vi "R2_Control.vi"() -> ()   [LabVIEW 2016]
uses:
  R2 Reactor Status v1.ctl
  Reactor Control/R1R2/R2/R2 SBR Mode Control.ctl
  Reactor Control/R1R2/R2/R2 pH Manual Control.ctl
  Reactor Control/R1R2/R2/R2 Pump Manual Control.ctl
  R2 DO Manual Control.ctl
  Reactor Control/R1R2/R2/R2Variables.lvlib
panel:
  out "Elapsed Time":dbl
  in  "Aerobic DO Control":T1={"DO set point (mg/L)"=1.5, "N2 Gain"=5.0, "Air Gain"=5.0, "DO Tolerance (mg/L)"=0.05, "Air Short Reaction Time (s)"=15.0, "Long Reaction Time (s)"=30.0, "N2 Short Reaction Time (s) 2"=10.0}
  out "pH and DO":cluster{"pH":dbl, "DO (mg/L)":dbl}(graph)
  out "DO Intercept":dbl
  out "DO Slope":dbl
  out "pH Intercept":dbl
  out "pH Slope":dbl
  in  "DO Control":T2
  in  "Reactor 2 Pumps Manual Control":T3
  in  "pH Control":T4
  in  "pH Control":T5={" pH Set Point"=7.5, " pH Tolerance"=0.1, "Reaction Time (s)"=15.0, "Pump On Time (s)"=3.0}
  in  "SBR Timing":T6={"Anaerobic Feed"=60.0, "Aerobic"=240.0, "Settle 1"=3.0, "Decant 1"=0.5, "Mix 2"=1.0, "Floc Effluent"=3.0, "Aerobic no DO control "=2.0, "Settle 2 (min)"=2.0, "Decant 2"=0.5, "Mix 3"=1.0, "Settle 3"=1.0, "Decant 3"=1.0, "Floc Return"=0.0}
  out "N2 and Air Flow":cluster{"N2 Flow":dbl, "Air Flow":dbl}(graph)
  out "Reactor 2 Status":T7 {"Compressed Air" format="%#.0g"; "Release Flow" format="%#.0g"; "DO Amp (A)" format="%#.4g"; "pH Amp (A)" format="%#.4g"; "DO (mg/L)" format="%#.2g"; "pH" format="%#.2g"}
  in  "Pumps Manual Control":bool
  in  "DO Manual Control":bool
  in  "pH Manual Control":bool
  in  "DO Calibrate":bool
  in  "pH Calibrate":bool
  # "On: Manual Mode\nOff: SBR Mode"
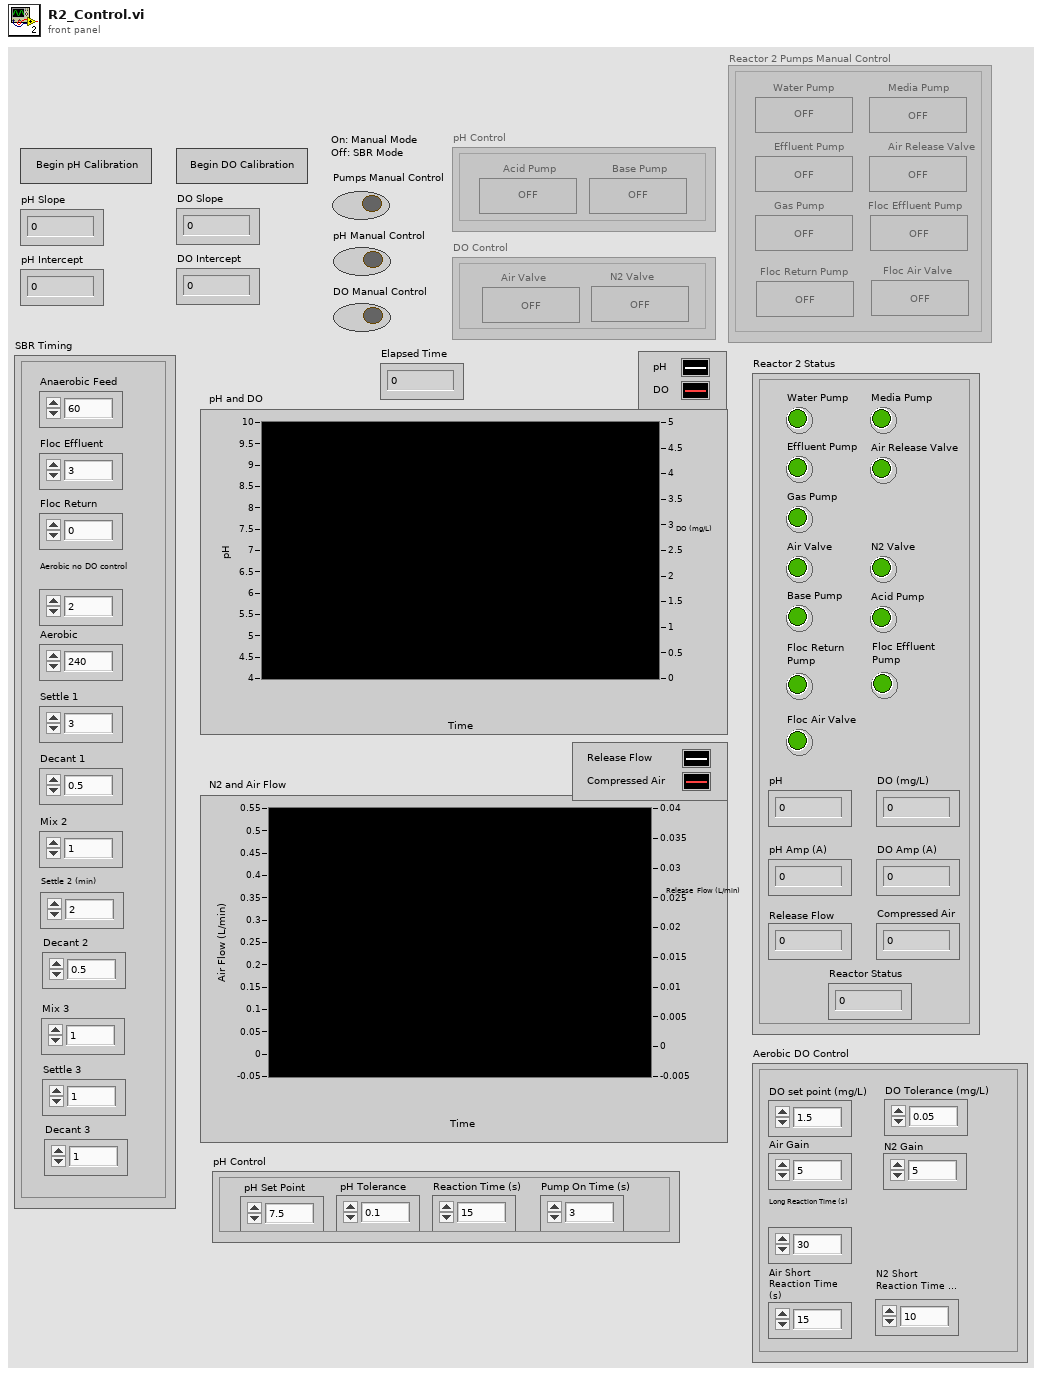
[diagram p1: front panel]
types:
  T1 = cluster{"DO set point (mg/L)":dbl, "N2 Gain":dbl, "Air Gain":dbl, "DO Tolerance (mg/L)":dbl, "Air Short Reaction Time (s)":dbl, "Long Reaction Time (s)":dbl, "N2 Short Reaction Time (s) 2":dbl}
  T2 = typedef "R2Variables.lvlib/R2 DO Manual Control.ctl" = cluster{"Air Valve":bool, "N2 Valve":bool}
  T3 = typedef "R2Variables.lvlib/R2 Pump Manual Control.ctl" = cluster{"Water Pump":bool, "Effluent Pump":bool, "Media Pump":bool, "Gas Pump":bool, "Air Release Valve":bool, "Floc Effluent Pump":bool, "Floc Return Pump":bool, "Floc Air Valve":bool}
  T4 = typedef "R2Variables.lvlib/R2 pH Manual Control.ctl" = cluster{"Acid Pump":bool, "Base Pump":bool}
  T5 = cluster{" pH Set Point":dbl, " pH Tolerance":dbl, "Reaction Time (s)":dbl, "Pump On Time (s)":dbl}
  T6 = typedef "R2Variables.lvlib/R2 SBR Mode Control.ctl" = cluster{"Anaerobic Feed":dbl, "Aerobic":dbl, "Settle 1":dbl, "Decant 1":dbl, "Mix 2":dbl, "Floc Effluent":dbl, "Aerobic no DO control ":dbl, "Settle 2 (min)":dbl, "Decant 2":dbl, "Mix 3":dbl, "Settle 3":dbl, "Decant 3":dbl, "Floc Return":dbl}
  T7 = typedef "R2Variables.lvlib/R2 Reactor Status v1.ctl" = cluster{"Water Pump":bool, "Media Pump":bool, "Effluent Pump":bool, "Base Pump":bool, "Gas Pump":bool, "Acid Pump":bool, "Air Release Valve":bool, "N2 Valve":bool, "pH":dbl, "DO (mg/L)":dbl, "pH Amp (A)":dbl, "DO Amp (A)":dbl, "Release Flow":dbl, "Compressed Air":dbl, "Reactor Status":sgl, "Air Valve":bool, "Floc Return \nPump":bool, "Floc Effluent\nPump ":bool, "Floc Air Valve":bool}
  T8 = enum8{"Enabled", "Disabled", "Disabled and Grayed Out"}
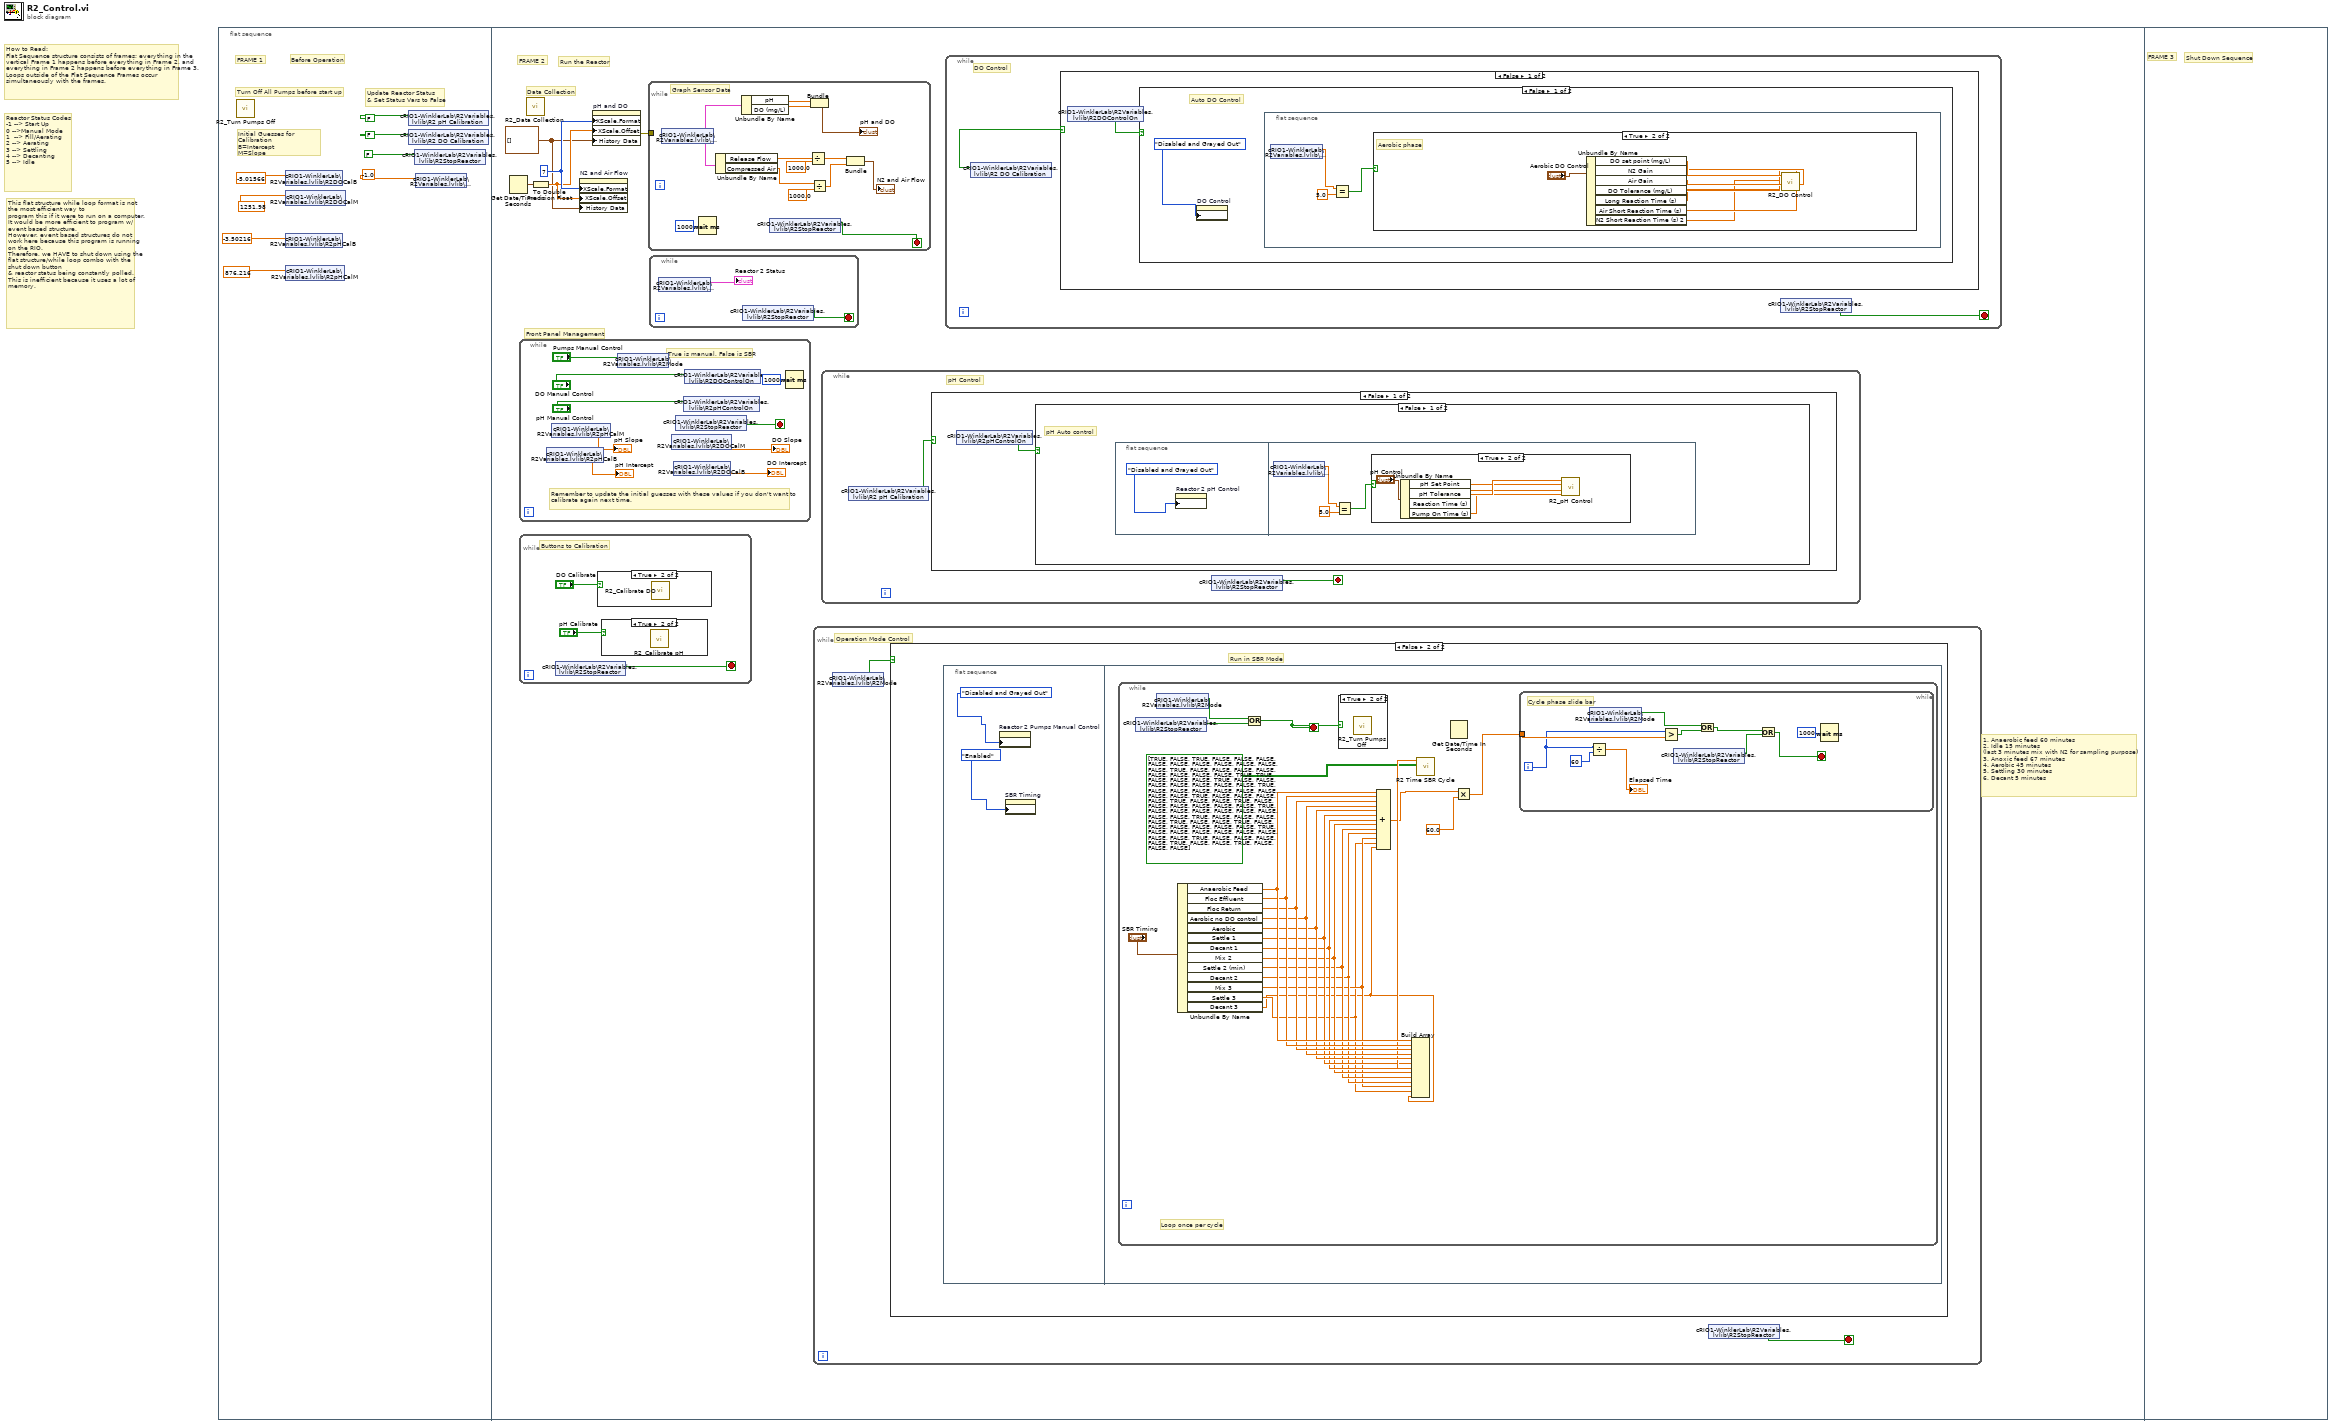
[diagram p0: block diagram]
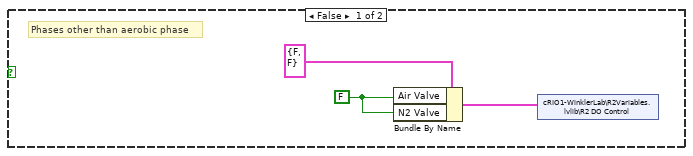
[diagram p2: hidden frame]
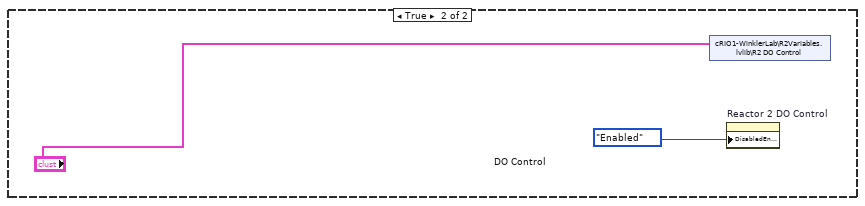
[diagram p3: hidden frame]
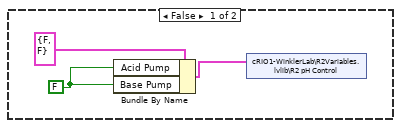
[diagram p7: hidden frame]
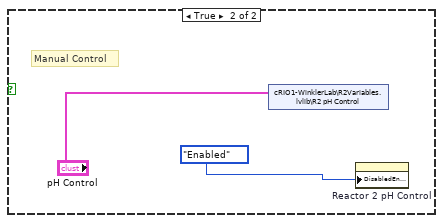
[diagram p8: hidden frame]
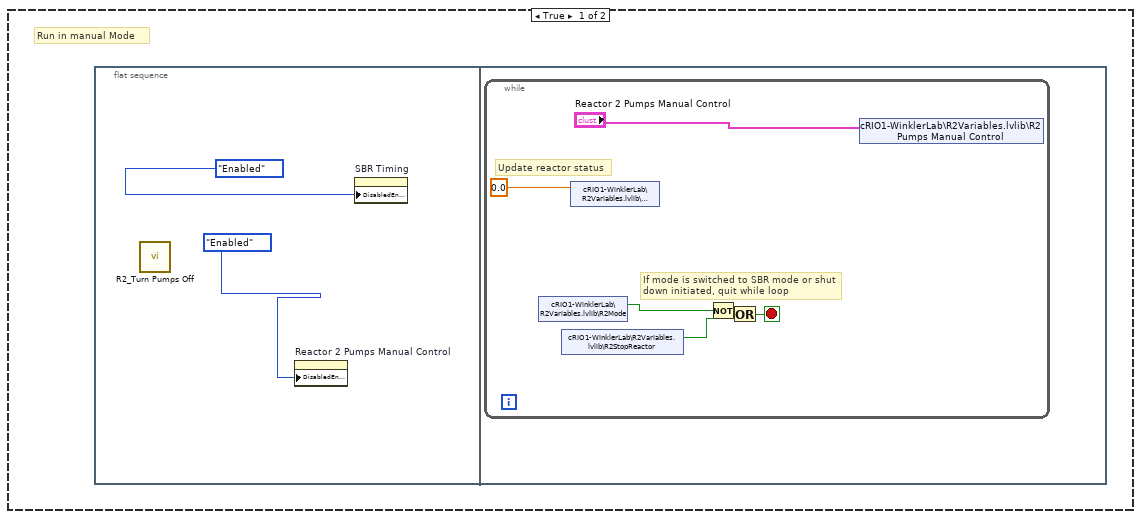
[diagram p10: hidden frame]
diagram:
  # "Reactor Status Codes\n-1 --> Start Up\n0 -->Manual Mode\n1  --> Fill/Aerating\n2 --> Aerating\n3 --> Settling\n4 --> Decanting\n5 --> Idle"
  # "How to Read:\nFlat Sequence structure consists of frames; everything in the vertical Frame 1 happens before everything in Frame 2, and everything in Frame 2 happens before everything in Frame 3.\nLoops outside of the Flat Sequence Frames occur simultaneously with the frames."
  # "This flat structure while loop format is not the most efficient way to \nprogram this if it were to run on a computer.\nIt would be more efficient to program w/ event based structure.\nHowever, event based structures do not work here because this program is running on the RIO.\nTherefore, we HAVE to shut down using the flat structure/while loop combo with the shut down button \n& reactor status being constantly polled.\nThis is inefficient because it uses a lot of memory."
  n1 = flat-sequence {
    frame #0 {
      # "Initial Guesses for Calibration\nB=Intercept\nM=Slope"
      # "Update Reactor Status \n& Set Status Vars to False"
      # "Turn Off All Pumps before start up"
      # "FRAME 1"
      # "Before Operation"
      n2 = call "R2_Turn Pumps Off.vi"() -> ()  [unwired: 12 in]
      n3 = shared-variable "cRIO1-WinklerLab\\R2Variables.lvlib\\R2DOCalB"(-5.01566 ("R1DOxCalB")) -> ()  [unwired: 1 in, 1 out]
      n4 = shared-variable "cRIO1-WinklerLab\\R2Variables.lvlib\\R2DOCalM"(1251.98 ("R1DOxCalM")) -> ()  [unwired: 1 in, 1 out]
      n5 = shared-variable "cRIO1-WinklerLab\\R2Variables.lvlib\\R2pHCalB"(-3.50216 ("R1pHCalB")) -> ()  [unwired: 1 in, 1 out]
      n6 = shared-variable "cRIO1-WinklerLab\\R2Variables.lvlib\\R2pHCalM"(876.216 ("R1pHCalM")) -> ()  [unwired: 1 in, 1 out]
      n7 = shared-variable "cRIO1-WinklerLab\\R2Variables.lvlib\\R2 pH Calibration"(FALSE ("pH Calibration")) -> ()  [unwired: 1 in, 1 out]
      n8 = shared-variable "cRIO1-WinklerLab\\R2Variables.lvlib\\R2 DO Calibration"(FALSE ("DO Calibration")) -> ()  [unwired: 1 in, 1 out]
      n9 = shared-variable "cRIO1-WinklerLab\\R2Variables.lvlib\\R2StopReactor"(FALSE ("R1Stop Reactor")) -> ()  [unwired: 1 in, 1 out]
      n10 = shared-variable "cRIO1-WinklerLab\\R2Variables.lvlib\\R2Phase"(-1.0) -> ()  [unwired: 1 in, 1 out]
    }
    frame #1 {
      w9 = cluster{"pH":dbl, "DO (mg/L)":dbl}[] [] ("History Data")
      w11 = u8 7 ("X Scale.Display Format:Format")
      # "1. Anaerobic feed 60 minutes\n2. Idle 15 minutes \n(last 3 minutes mix with N2 for sampling purpose)\n3. Anoxic feed 67 minutes\n4. Aerobic 45 minutes\n5. Settling 30 minutes\n6. Decant 5 minutes"
      # "Front Panel Management"
      # "Data Collection"
      # "FRAME 2"
      # "Run the Reactor"
      n11 = Get Date/Time In Seconds() -> (seconds since 1Jan1904=w13:timestamp)
      n12 = while {
        stop <- w73 stop-if-true
        # "Remember to update the initial guesses with these values if you don't want to calibrate again next time."
        # "True is manual, False is SBR"
        n13 = shared-variable "cRIO1-WinklerLab\\R2Variables.lvlib\\R2pHCalB"() -> (→"pH Intercept":dbl)  [unwired: 1 in, 1 out]
        n14 = shared-variable "cRIO1-WinklerLab\\R2Variables.lvlib\\R2pHCalM"() -> (→"pH Slope":dbl)  [unwired: 1 in, 1 out]
        n15 = shared-variable "cRIO1-WinklerLab\\R2Variables.lvlib\\R2Mode"("Pumps Manual Control") -> ()  [unwired: 1 in, 1 out]
        n16 = shared-variable "cRIO1-WinklerLab\\R2Variables.lvlib\\R2DOCalM"() -> (→"DO Slope":dbl)  [unwired: 1 in, 1 out]
        n17 = shared-variable "cRIO1-WinklerLab\\R2Variables.lvlib\\R2DOCalB"() -> (→"DO Intercept":dbl)  [unwired: 1 in, 1 out]
        n18 = shared-variable "cRIO1-WinklerLab\\R2Variables.lvlib\\R2StopReactor"() -> (w73:bool)  [unwired: 1 in, 1 out]
        n19 = shared-variable "cRIO1-WinklerLab\\R2Variables.lvlib\\R2pHControlOn"("pH Manual Control") -> ()  [unwired: 1 in, 1 out]
        n20 = shared-variable "cRIO1-WinklerLab\\R2Variables.lvlib\\R2DOControlOn"("DO Manual Control") -> ()  [unwired: 1 in, 1 out]
        n21 = Wait (ms)(milliseconds to wait=u32 1000) -> ()  [unwired: 1 out]
      }
      n22 = while {
        stop <- w49 stop-if-true
        # "Buttons to Calibration"
        n23 = shared-variable "cRIO1-WinklerLab\\R2Variables.lvlib\\R2StopReactor"() -> (w49:bool)  [unwired: 1 in, 1 out]
        n24 = case shown="True" "DO Calibrate" {
          frame False {
          }
          frame True {
            n25 = call "R2_Calibrate DO.vi"() -> ()  [unwired: 12 in]
          }
        }
        n26 = case shown="True" "pH Calibrate" {
          frame False {
          }
          frame True {
            n27 = call "R2_Calibrate pH.vi"() -> ()  [unwired: 12 in]
          }
        }
      }
      n28 = call "R2_Data Collection.vi"() -> ()  [unwired: 12 in]
      n29 = To Double Precision Float(number=w13) -> (double precision float=w10:dbl)
      n30 = property on="N2 and Air Flow" class="WFChart (strict)"("XScale.Format"=w11, "XScale.Offset"=w10, "History Data"=w9) -> ()  [unwired: 2 in, 2 out]
      n31 = property on="pH and DO" class="WFChart (strict)"("XScale.Format"=w11, "XScale.Offset"=w10, "History Data"=w9) -> (error out=w12:errorcluster)  [unwired: 2 in, 1 out]
      n32 = while {
        tunnel: w12 -> [_]
        stop <- w24 stop-if-true
        # "Graph Sensor Data"
        n33 = shared-variable "cRIO1-WinklerLab\\R2Variables.lvlib\\R2Status"() -> (w25:T7)  [unwired: 1 in, 1 out]
        n34 = Wait (ms)(milliseconds to wait=u32 1000) -> ()  [unwired: 1 out]
        n35 = Unbundle By Name(w25) -> ("Release Flow"=w21:dbl, "Compressed Air"=w18:dbl)
        n36 = Unbundle By Name(w25) -> ("pH"=w26:dbl, "DO (mg/L)"=w27:dbl)
        n37 = shared-variable "cRIO1-WinklerLab\\R2Variables.lvlib\\R2StopReactor"() -> (w24:bool)  [unwired: 1 in, 1 out]
        n38 = Divide(x=w21, y=1000.0) -> (x/y=w17:dbl)
        n39 = Bundle("pH"=w26, "DO (mg/L)"=w27) -> (→"pH and DO":cluster{"pH":dbl, "DO (mg/L)":dbl})  [unwired: 1 in]
        n40 = Divide(x=w18, y=1000.0) -> (x/y=w16:dbl)
        n41 = Bundle(w17, w16) -> (→"N2 and Air Flow":cluster{dbl, dbl})  [unwired: 1 in]
      }
      n42 = while {
        stop <- w14 stop-if-true
        n43 = shared-variable "cRIO1-WinklerLab\\R2Variables.lvlib\\R2Status"() -> (→"Reactor 2 Status":T7)  [unwired: 1 in, 1 out]
        n44 = shared-variable "cRIO1-WinklerLab\\R2Variables.lvlib\\R2StopReactor"() -> (w14:bool)  [unwired: 1 in, 1 out]
      }
      n45 = while {
        stop <- w79 stop-if-true
        # "Operation Mode Control"
        n46 = shared-variable "cRIO1-WinklerLab\\R2Variables.lvlib\\R2Mode"() -> (w78:bool)  [unwired: 1 in, 1 out]
        n47 = case shown="False" w78 {
          frame True {
            # "Run in manual Mode"
            n48 = flat-sequence {
              frame #0 {
                n49 = call "R2_Turn Pumps Off.vi"() -> ()  [unwired: 12 in]
                n50 = property on="Reactor 2 Pumps Manual Control" class="Clust (strict)"("DisabledEnum"=T8."Enabled" ("Disabled")) -> ()  [unwired: 2 in, 2 out]
                n51 = property on="SBR Timing" class="Clust (strict)"("DisabledEnum"=T8."Enabled" ("Disabled")) -> ()  [unwired: 2 in, 2 out]
              }
              frame #1 {
                n52 = while {
                  stop <- w86 stop-if-true
                  # "If mode is switched to SBR mode or shut \ndown initiated, quit while loop"
                  # "Update reactor status"
                  n53 = shared-variable "cRIO1-WinklerLab\\R2Variables.lvlib\\R2Mode"() -> (w84:bool)  [unwired: 1 in, 1 out]
                  n54 = shared-variable "cRIO1-WinklerLab\\R2Variables.lvlib\\R2StopReactor"() -> (w83:bool)  [unwired: 1 in, 1 out]
                  n55 = shared-variable "cRIO1-WinklerLab\\R2Variables.lvlib\\R2Phase"(0.0 ("Reactor Status")) -> ()  [unwired: 1 in, 1 out]
                  n56 = Not(x=w84) -> (.not. x?=w87:bool)
                  n57 = Or(x=w87, y=w83) -> (x .or. y?=w86:bool)
                  n58 = shared-variable "cRIO1-WinklerLab\\R2Variables.lvlib\\R2 Pumps Manual Control"("Reactor 2 Pumps Manual Control") -> ()  [unwired: 1 in, 1 out]
                }
              }
            }
          }
          frame False {
            # "Run in SBR Mode"
            n59 = flat-sequence {
              frame #0 {
                n60 = property on="Reactor 2 Pumps Manual Control" class="Clust (strict)"("DisabledEnum"=T8."Disabled and Grayed Out" ("Disabled")) -> ()  [unwired: 2 in, 2 out]
                n61 = property on="SBR Timing" class="Clust (strict)"("DisabledEnum"=T8."Enabled" ("Disabled")) -> ()  [unwired: 2 in, 2 out]
              }
              frame #1 {
                n62 = while {
                  stop <- w111 stop-if-true
                  # "Loop once per cycle"
                  n63 = shared-variable "cRIO1-WinklerLab\\R2Variables.lvlib\\R2StopReactor"() -> (w109:bool)  [unwired: 1 in, 1 out]
                  n64 = shared-variable "cRIO1-WinklerLab\\R2Variables.lvlib\\R2Mode"() -> (w110:bool)  [unwired: 1 in, 1 out]
                  n65 = Unbundle By Name("SBR Timing") -> ("Anaerobic Feed"=w107:dbl, "Floc Effluent"=w106:dbl, "Floc Return"=w105:dbl, "Aerobic no DO control"=w104:dbl, "Aerobic"=w103:dbl, "Settle 1"=w97:dbl, "Decant 1"=w96:dbl, "Mix 2"=w95:dbl, "Settle 2 (min)"=w94:dbl, "Decant 2"=w93:dbl, "Mix 3"=w92:dbl, "Settle 3"=w91:dbl, "Decant 3"=w90:dbl)
                  n66 = Or(x=w110, y=w109) -> (x .or. y?=w111:bool)
                  n67 = case shown="True" w111 {
                    frame False {
                    }
                    frame True {
                      n68 = call "R2_Turn Pumps Off.vi"() -> ()  [unwired: 12 in]
                    }
                  }
                  n69 = Compound Arithmetic op=ADD(w107, w106, w105, w104, w103, w97, w96, w95, w94, w93, w92, w91, w90) -> (w98:dbl)
                  n70 = Build Array(w107, w106, w105, w104, w103, w97, w96, w95, w94, w93, w92, w91, w90) -> (w102:dbl[])
                  n71 = call "R2 Time SBR Cycle.vi"("Pump Status Array"=bool[][] [[TRUE, FALSE, TRUE, FALSE, FALSE, FALSE, FALSE, FALSE], [FALSE, FALSE, FALSE, FALSE, FALSE, TRUE, FALSE, FALSE], [FALSE, FALSE, FALSE, FALSE, FALSE, FALSE, TRUE, TRUE], [FALSE, FALSE, FALSE, TRUE, FALSE, FALSE, FALSE, FALSE], [FALSE, FALSE, FALSE, TRUE, FALSE, FALSE, FALSE, FALSE], [FALSE, FALSE, FALSE, FALSE, TRUE, FALSE, FALSE, FALSE], [FALSE, TRUE, FALSE, FALSE, TRUE, FALSE, FALSE, FALSE], [FALSE, FALSE, FALSE, TRUE, FALSE, FALSE, FALSE, FALSE], [FALSE, FALSE, FALSE, FALSE, TRUE, FALSE, FALSE, FALSE], [FALSE, TRUE, FALSE, FALSE, TRUE, FALSE, FALSE, FALSE], [FALSE, FALSE, FALSE, TRUE, FALSE, FALSE, FALSE, FALSE], [FALSE, FALSE, FALSE, FALSE, TRUE, FALSE, FALSE, FALSE], [FALSE, TRUE, FALSE, FALSE, TRUE, FALSE, FALSE, FALSE]], "Array"=w102) -> ()  [unwired: 10 in]
                  n72 = Get Date/Time In Seconds() -> ()  [unwired: 1 out]
                  n73 = Multiply(x=w98, y=60.0) -> (x*y=w99:dbl)
                  n74 = while {
                    tunnel: w99 -> [w120]
                    i -> [w113]
                    stop <- w114 stop-if-true
                    # "Cycle phase slide bar"
                    n75 = shared-variable "cRIO1-WinklerLab\\R2Variables.lvlib\\R2Mode"() -> (w117:bool)  [unwired: 1 in, 1 out]
                    n76 = Divide(x=w113, y=60) -> (x/y=→"Elapsed Time":dbl)
                    n77 = Greater?(x=w113, y=w120) -> (0:w118:bool)
                    n78 = shared-variable "cRIO1-WinklerLab\\R2Variables.lvlib\\R2StopReactor"() -> (w115:bool)  [unwired: 1 in, 1 out]
                    n79 = Or(x=w117, y=w118) -> (x .or. y?=w116:bool)
                    n80 = Or(x=w116, y=w115) -> (x .or. y?=w114:bool)
                    n81 = Wait (ms)(milliseconds to wait=u32 1000) -> ()  [unwired: 1 out]
                  }
                }
              }
            }
          }
        }
        n82 = shared-variable "cRIO1-WinklerLab\\R2Variables.lvlib\\R2StopReactor"() -> (w79:bool)  [unwired: 1 in, 1 out]
      }
      n83 = while {
        stop <- w53 stop-if-true
        # "pH Control"
        n84 = shared-variable "cRIO1-WinklerLab\\R2Variables.lvlib\\R2 pH Calibration"() -> (w52:bool)  [unwired: 1 in, 1 out]
        n85 = case shown="False" w52 {
          frame False {
            n86 = shared-variable "cRIO1-WinklerLab\\R2Variables.lvlib\\R2pHControlOn"() -> (w54:bool)  [unwired: 1 in, 1 out]
            n87 = case shown="False" w54 {
              frame False {
                # "pH Auto control"
                n88 = flat-sequence {
                  frame #0 {
                    n89 = property on="Reactor 2 pH Control" class="Clust (strict)"("DisabledEnum"=T8."Disabled and Grayed Out" ("Disabled")) -> ()  [unwired: 2 in, 2 out]
                  }
                  frame #1 {
                    n90 = shared-variable "cRIO1-WinklerLab\\R2Variables.lvlib\\R2Phase"() -> (w58:dbl)  [unwired: 1 in, 1 out]
                    n91 = Equal?(x=w58, y=5.0) -> (x = y?=w56:bool)
                    n92 = case shown="True" w56 {
                      frame False {
                        w60 = FALSE
                        n93 = Bundle By Name(cluster=T4 {"Acid Pump"=FALSE, "Base Pump"=FALSE} ("Reactor 2 pH Control"), "Acid Pump"=w60, "Base Pump"=w60) -> (w59:T4)
                        n94 = shared-variable "cRIO1-WinklerLab\\R2Variables.lvlib\\R2 pH Control"(w59) -> ()  [unwired: 1 in, 1 out]
                      }
                      frame True {
                        n95 = Unbundle By Name("pH Control") -> ("pH Set Point"=w64:dbl, "pH Tolerance"=w65:dbl, "Reaction Time (s)"=w63:dbl, "Pump On Time (s)"=w62:dbl)
                        n96 = call "R2_pH Control.vi"("Pump On Time (s)"=w62, "Reaction Time (s)"=w63, "pH Set Point"=w64, "pH Tolerance"=w65) -> ()  [unwired: 8 in]
                      }
                    }
                  }
                }
              }
              frame True {
                # "Manual Control"
                n97 = shared-variable "cRIO1-WinklerLab\\R2Variables.lvlib\\R2 pH Control"("pH Control") -> ()  [unwired: 1 in, 1 out]
                n98 = property on="Reactor 2 pH Control" class="Clust (strict)"("DisabledEnum"=T8."Enabled" ("Disabled")) -> ()  [unwired: 2 in, 2 out]
              }
            }
          }
          frame True {
          }
        }
        n99 = shared-variable "cRIO1-WinklerLab\\R2Variables.lvlib\\R2StopReactor"() -> (w53:bool)  [unwired: 1 in, 1 out]
      }
      n100 = while {
        stop <- w30 stop-if-true
        # "DO Control"
        n101 = shared-variable "cRIO1-WinklerLab\\R2Variables.lvlib\\R2 DO Calibration"() -> (w29:bool)  [unwired: 1 in, 1 out]
        n102 = case shown="False" w29 {
          frame False {
            n103 = shared-variable "cRIO1-WinklerLab\\R2Variables.lvlib\\R2DOControlOn"() -> (w31:bool)  [unwired: 1 in, 1 out]
            n104 = case shown="False" w31 {
              frame False {
                # "Auto DO Control"
                n105 = property on="DO Control" class="Clust (strict)"("DisabledEnum"=T8."Disabled and Grayed Out" ("Disabled")) -> ()  [unwired: 2 in, 2 out]
                n106 = flat-sequence {
                  frame #0 {
                    n107 = shared-variable "cRIO1-WinklerLab\\R2Variables.lvlib\\R2Phase"() -> (w35:dbl)  [unwired: 1 in, 1 out]
                    n108 = Equal?(x=w35, y=5.0) -> (x = y?=w33:bool)
                    n109 = case shown="True" w33 {
                      frame False {
                        w37 = FALSE
                        # "Phases other than aerobic phase"
                        n110 = Bundle By Name(cluster=T2 {"Air Valve"=FALSE, "N2 Valve"=FALSE} ("Reactor 2 DO Control"), "Air Valve"=w37, "N2 Valve"=w37) -> (w38:T2)
                        n111 = shared-variable "cRIO1-WinklerLab\\R2Variables.lvlib\\R2 DO Control"(w38) -> ()  [unwired: 1 in, 1 out]
                      }
                      frame True {
                        # "Aerobic phase"
                        n112 = Unbundle By Name("Aerobic DO Control") -> ("DO set point (mg/L)"=w45:dbl, "N2 Gain"=w44:dbl, "Air Gain"=w43:dbl, "DO Tolerance (mg/L)"=w42:dbl, "Long Reaction Time (s)"=w41:dbl, "Air Short Reaction Time (s)"=w40:dbl, "N2 Short Reaction Time (s) 2"=w39:dbl)
                        n113 = call "R2_DO Control.vi"("Air Short Reaction Time (s)"=w40, "N2 Gain"=w44, "DO Tolerance (mg/L)"=w42, "Long Reaction Time (s)"=w41, "Air Gain"=w43, "N2 Short Reaction Time (s)"=w39, "DO Set Point (mg/L)"=w45) -> ()  [unwired: 1 in]
                      }
                    }
                  }
                }
              }
              frame True {
                n114 = shared-variable "cRIO1-WinklerLab\\R2Variables.lvlib\\R2 DO Control"("DO Control") -> ()  [unwired: 1 in, 1 out]
                n115 = property on="Reactor 2 DO Control" class="Clust (strict)"("DisabledEnum"=T8."Enabled" ("Disabled")) -> ()  [unwired: 2 in, 2 out]
              }
            }
          }
          frame True {
          }
        }
        n116 = shared-variable "cRIO1-WinklerLab\\R2Variables.lvlib\\R2StopReactor"() -> (w30:bool)  [unwired: 1 in, 1 out]
      }
    }
    frame #2 {
      # "FRAME 3"
      # "Shut Down Sequence"
    }
  }
